vi "UTL_Controller Running monitor.vi"(5 "Error In":errorcluster, 6 "Data":dbl[][][](array[numeric]), 7 "ReportPath":path, 9 "PyPath":path, 11 "ReportXlsxPath":path) -> (19 "Error Out":errorcluster)   [LabVIEW 2019]
uses:
  Variable global de carga.vi
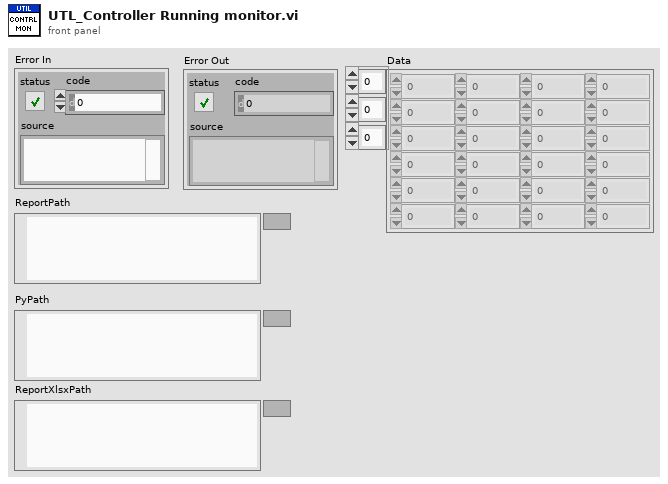
[diagram p1: front panel]
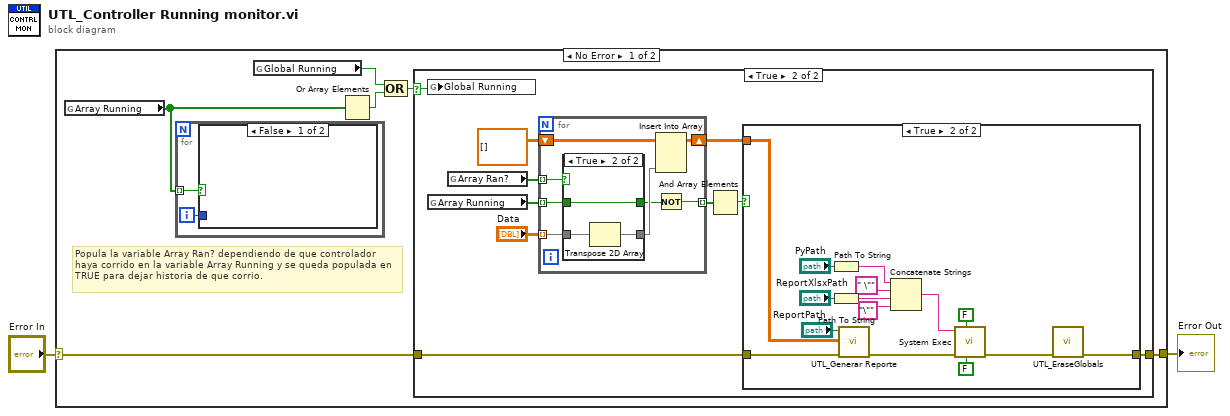
[diagram p0: block diagram]
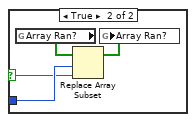
[diagram p2: hidden frame]
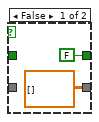
[diagram p4: hidden frame]
diagram:
  n1 = case shown="No Error" "Error In" {
    selector: "Error In" -> [w7 w55]
    tunnel: [w8 w55] -> w2
    frame No Error {
      # "Popula la variable Array Ran? dependiendo de que controlador haya corrido en la variable Array Running y se queda populada en TRUE para dejar historia de que corrio."
      n2 = global read "Variable global de carga.vi" "Array Running"() -> (w3:bool[])
      n3 = for {
        tunnel: w3 -> [w9] mode=indexing
        i -> [w10]
        n4 = case shown="False" w9 {
          selector: w9 -> [_ w13]
          tunnel: w10 -> [_ w14]
          frame False {
          }
          frame True {
            n5 = global read "Variable global de carga.vi" "Array Ran?"() -> (w11:bool[])
            n6 = Replace Array Subset(array=w11, new element=w13, index=w14) -> (w12:bool[])
            n7 = global write "Variable global de carga.vi" "Array Ran?"(w12) -> ()
          }
        }
      }
      n8 = global read "Variable global de carga.vi" "Global Running"() -> (w4:bool)
      n9 = Or Array Elements(Boolean array=w3) -> (logical OR=w6:bool)
      n10 = Compound Arithmetic op=OR(w4, w6) -> (w5:bool)
      n11 = case shown="True" w5 {
        selector: w5 -> [_ w24]
        tunnel: [w15 w25] -> w8
        tunnel: w7 -> [w15 w23]
        frame False {
        }
        frame True {
          n12 = global write "Variable global de carga.vi" "Global Running"(w24) -> ()
          n13 = global read "Variable global de carga.vi" "Array Running"() -> (w18:bool[])
          n14 = global read "Variable global de carga.vi" "Array Ran?"() -> (w19:bool[])
          n15 = for {
            tunnel: w19 -> [w33] mode=indexing
            tunnel: w18 -> [w31] mode=indexing
            tunnel: "Data" -> [w32] mode=indexing
            shift-right: [w29] -> w16
            shift-left: dbl[][] [] ("Results C2") -> [w30]
            tunnel: [w26] -> w21 mode=indexing
            n16 = case shown="True" w33 {
              tunnel: w32 -> [_ w37]
              tunnel: [dbl[][] [] ("Results C2") w36] -> w28
              tunnel: w31 -> [_ w38]
              tunnel: [FALSE w38] -> w27
              frame False {
              }
              frame True {
                n17 = Transpose 2D Array(2D array=w37) -> (transposed array=w36:dbl[][])
              }
            }
            n18 = Insert Into Array(array=w30, new element=w28) -> (w29:dbl[][])  [unwired: 2 in]
            n19 = Not(x=w27) -> (.not. x?=w26:bool)
          }
          n20 = And Array Elements(Boolean array=w21) -> (logical AND=w20:bool)
          n21 = case shown="True" w20 {
            tunnel: [w39 w46] -> w25
            tunnel: w23 -> [w39 w54]
            tunnel: w16 -> [_ w49]
            frame False {
            }
            frame True {
              n22 = Path To String(path="PyPath") -> (string=w44:string)
              n23 = Path To String(path="ReportXlsxPath") -> (string=w43:string)
              n24 = call "UTL_Generar Reporte.vi"("Error in"=w54, "Data"=w49, "Results Path"="ReportPath") -> ("Error out"=w52:errorcluster)  [unwired: 7 in, 1 out]
              n25 = Concatenate Strings(w44, " \"" ("string"), w43, "\"" ("string")) -> (w40:string)
              n26 = call <vilib>:"System Exec.vi"("run minimized? (F)"=FALSE, "wait until completion? (T)"=FALSE, "error in (no error)"=w52, "command line"=w40) -> ("error out"=w47:errorcluster)  [unwired: 4 in, 3 out]
              n27 = call "UTL_EraseGlobals.vi"("error in (no error)"=w47) -> ("error out"=w46:errorcluster)  [unwired: 10 in]
            }
          }
        }
      }
    }
    frame Error {
    }
  }
  "Error Out" <- w2
